vi "Open Config File.vi"(8 "error in (no error)":errorcluster, 10 "create file if necessary (T)":bool=TRUE, 11 "Process in":refnum<class "Process.lvclass">) -> (0 "error out":errorcluster, 1 "file created?":bool, 2 "refnum out":T1, 3 "Process out":refnum<class "Process.lvclass">)   [LabVIEW 2020, in "Configuration File.lvlib"]
doc: "High-level function for opening configuration file data from process class."
uses:
  Configuration File.lvlib
  Process Classes/Process/Process.lvclass
  <vilib>/Utility/config.llb/Config Data RefNum.ctl
  Process Classes/Process/Process.lvclass/Process.ctl
  <vilib>/Utility/config.llb/NI_LVConfig.lvlib
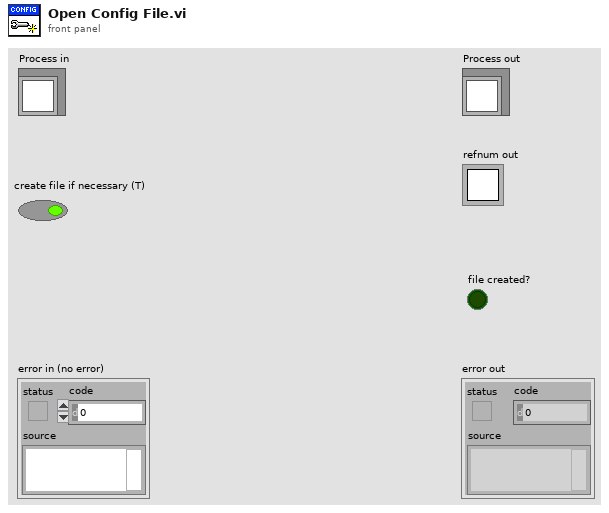
[diagram p1: front panel]
types:
  T1 = typedef "NI_LVConfig.lvlib/Config Data RefNum.ctl" = refnum<k1>
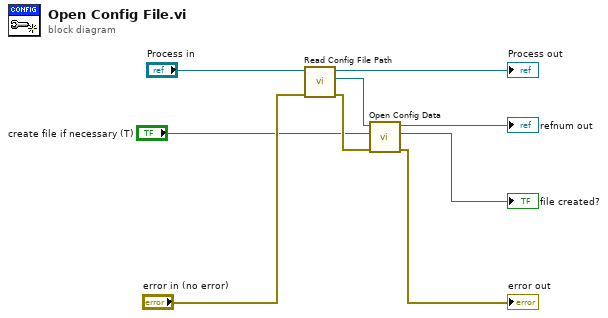
[diagram p0: block diagram]
diagram:
  n1 = call "Read Config File Path.vi"("error in (no error)"="error in (no error)", "Process In"="Process in") -> ("error out"=w6:errorcluster, "Config File Path"=w3:path, "Process Out"=→"Process out":refnum<class "Process.lvclass">)  [unwired: 7 in]
  n2 = call <vilib>:"Open Config Data.vi"("error in (no error)"=w6, "create file if necessary (T)"="create file if necessary (T)", "configuration file path"=w3) -> ("error out"=→"error out":errorcluster, "file created?"=→"file created?":bool, "refnum"=→"refnum out":T1)  [unwired: 6 in]
